vi "Test Display Panel V3.vi"() -> ()   [LabVIEW 2016, in "Display Panel.lvlib" / "Display Panel V3.lvclass"]
uses:
  Display Panel V3.lvclass
  C:/Users/Jlarrieux/Documents/LabView Git Repo/Generic Instrument/Subpanel Insertion/Subpanel Inserter.lvclass
  C:/Program Files (x86)/National Instruments/LabVIEW 2016/vi.lib/ActorFramework/Actor/Actor.lvclass
  Display Panel V3 Messages/Insert into SubPanel Msg/Insert into SubPanel Msg.lvclass/Insert into SubPanel Msg.ctl
  <vilib>/ActorFramework/Message Enqueuer/Message Enqueuer.lvclass/Message Enqueuer.ctl
  <vilib>/ActorFramework/Message Enqueuer/Enqueue.vi
  Display Panel V3 Messages/Insert into SubPanel Msg/Insert into SubPanel Msg.lvclass
  C:/Program Files (x86)/National Instruments/LabVIEW 2016/vi.lib/ActorFramework/Message/Message.lvclass
  <vilib>/ActorFramework/Stop Msg/Stop Msg.lvclass
  <vilib>/ActorFramework/Message Priority Queue/Priority Enqueue.vi
  <vilib>/ActorFramework/Actor/Actor.lvclass
panel:
  out "error out 4":errorcluster
  out "error out 3":errorcluster
  out "error out 2":errorcluster
  out "error out":errorcluster
  out "Numeric Control":i32
  in  "Boolean":bool=TRUE
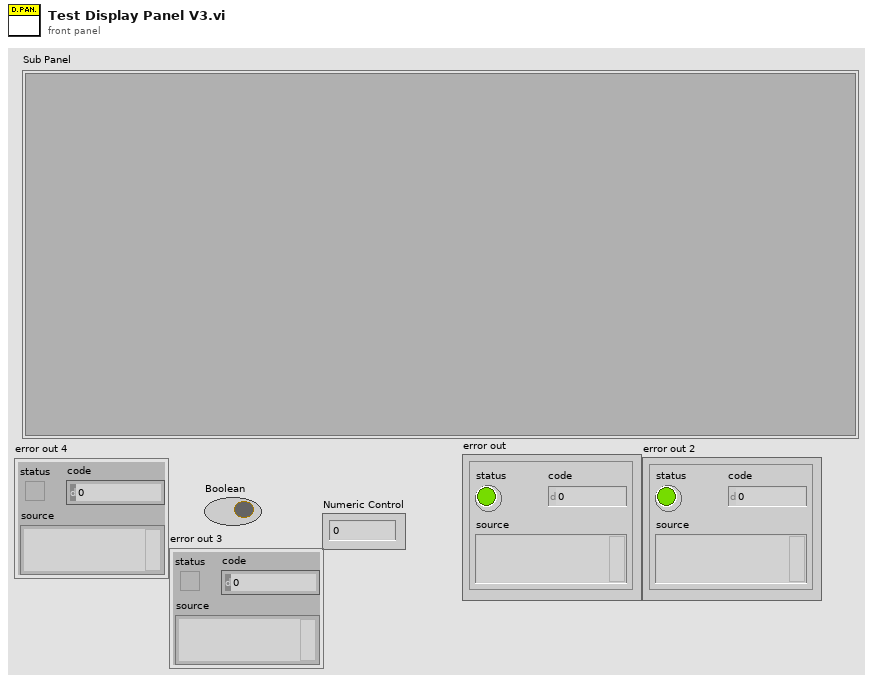
[diagram p1: front panel]
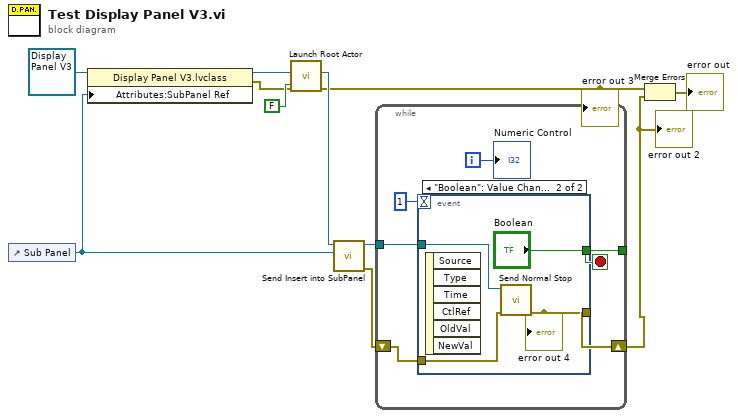
[diagram p0: block diagram]
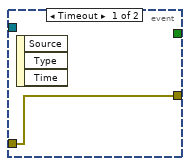
[diagram p2: hidden frame]
diagram:
  n1 = control-ref of="Sub Panel"() -> (w6:refnum<vi>)
  n2 = property class="Display Panel V3.lvclass"(reference=refnum<class "Display Panel V3.lvclass"> refnum ("Display Panel.lvlib:Display Panel V3.lvclass"), "Attributes:SubPanel Ref"=w6) -> (reference out=w9:refnum<class "Display Panel V3.lvclass">, error out=w8:errorcluster)  [unwired: 1 in]
  n3 = call <vilib>:"Launch Root Actor.vi"("Open Actor Core front panel? (F)"=FALSE, "error in (no error)"=w8, "Actor"=w9) -> ("error out"=w4:errorcluster, "Actor's Enqueuer"=w7:refnum<class "Message Enqueuer.lvclass">)  [unwired: 7 in]
  "error out 3" <- w4
  n4 = call "Send Insert into SubPanel.vi"("SubPanel Ref"=w6, "Message Enqueuer"=w7) -> ("error out"=w2:errorcluster, "Message Enqueuer out"=w5:refnum<class "Message Enqueuer.lvclass">)  [unwired: 8 in]
  n5 = while {
    tunnel: [w15] -> _
    tunnel: w5 -> [w14]
    shift-right: [w12] -> w1
    shift-left: w2 -> [w13]
    i -> [w17]
    stop <- w15 stop-if-true
    n6 = event shown="[1] \"Boolean\": Value Change" {
      selector: _ -> [_ _]
      dyn-events: _ -> [_ _]
      timeout: 1 -> [_ _]
      tunnel: [_ "Boolean"] -> w15
      tunnel: w14 -> [_ w21]
      tunnel: [w18 w20] -> w12
      tunnel: w13 -> [w18 w19]
      event Timeout {
        n7 = event-data() -> ()  [unwired: 1 in, 3 out]
      }
      event "Boolean": Value Change {
        n8 = event-data() -> ()  [unwired: 1 in, 6 out]
        n9 = call <vilib>:"Send Normal Stop.vi"("error in (no error)"=w19, "Message Enqueuer"=w21) -> ("error out"=w20:errorcluster)  [unwired: 9 in]
        "error out 4" <- w20
      }
    }
    "Numeric Control" <- w17
  }
  "error out 2" <- w1
  n10 = Merge Errors(w4, w1) -> (→"error out":errorcluster)
